vi "flat secuence local.vi"() -> ()   [LabVIEW 2020]
panel:
  out "String 2":string
  out "Boolean 2":bool
  out "Numeric":dbl
  in  "String":string
  in  "Boolean":bool
  in  "Thermometer 2":dbl(slide) scale=0.0..100.0
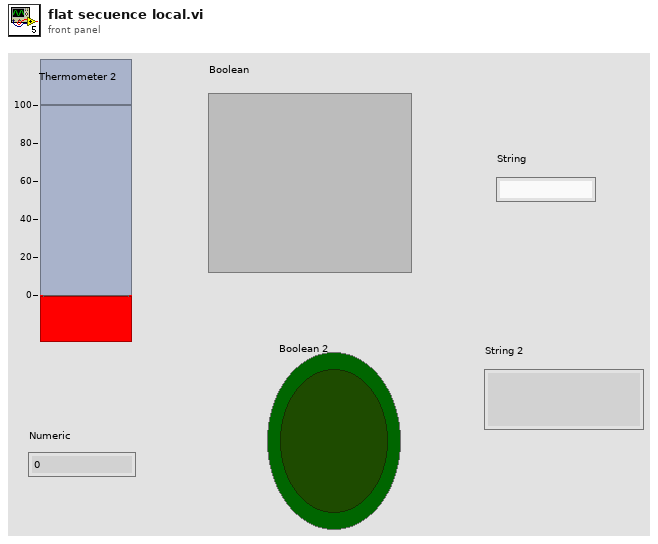
[diagram p1: front panel]
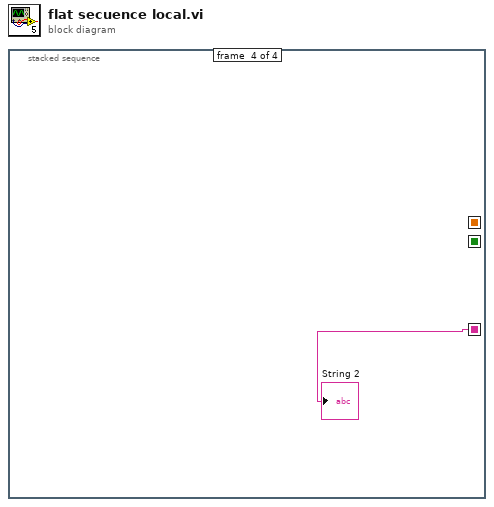
[diagram p0: block diagram]
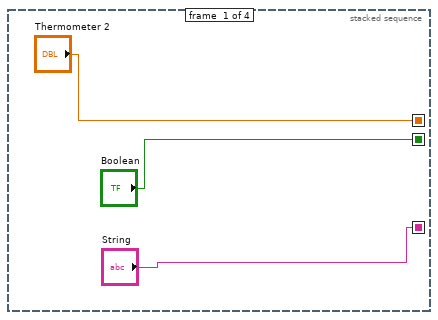
[diagram p2: hidden frame]
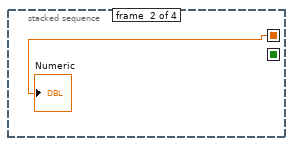
[diagram p3: hidden frame]
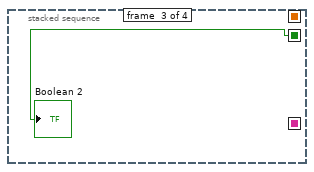
[diagram p4: hidden frame]
diagram:
  n1 = stacked-sequence {
    seq-local: ["Thermometer 2" _ _ _] -> [_ w4 _ _]
    seq-local: ["Boolean" _ _ _] -> [_ _ w5 _]
    seq-local: ["String" _ _ _] -> [_ _ _ w6]
    frame #0 {
    }
    frame #1 {
      "Numeric" <- w4
    }
    frame #2 {
      "Boolean 2" <- w5
    }
    frame #3 {
      "String 2" <- w6
    }
  }
